vi "sub_scout_cmd-pacekt-conversion.vi"(8 "Frame ID":u8, 10 "Angular Velocity":dbl, 11 "Linear Velocity":dbl) -> (2 "CMD":u8[](array[numeric]))   [LabVIEW 2019]
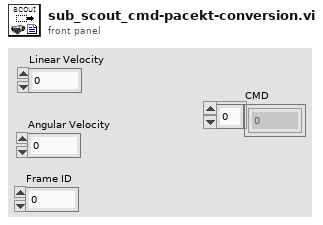
[diagram p1: front panel]
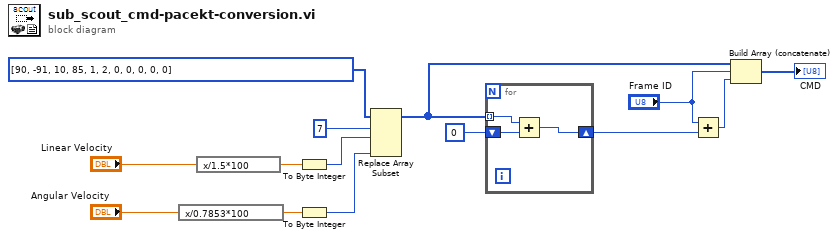
[diagram p0: block diagram]
diagram:
  n1 = expression code="x/0.7853*100"("Angular Velocity") -> (w2:dbl)
  n2 = expression code="x/1.5*100"("Linear Velocity") -> (w5:dbl)
  n3 = To Byte Integer(number=w5) -> (8bit integer=w4:i8)
  n4 = To Byte Integer(number=w2) -> (8bit integer=w1:i8)
  n5 = Replace Array Subset(array=i8[] [90, -91, 10, 85, 1, 2, 0, 0, 0, 0, 0] ("unsigned byte array"), new element #1=w4, index #1=7 ("index"), new element #2=w1) -> (w7:i8[])  [unwired: 1 in]
  n6 = for {
    tunnel: w7 -> [w17] mode=indexing
    shift-right: [w15] -> w13
    shift-left: u8 0 -> [w16]
    n7 = Add(x=w17, y=w16) -> (x+y=w15:u8)
  }
  n8 = Add(x="Frame ID", y=w13) -> (x+y=w11:u8)
  n9 = Build Array (concatenate)(w7, "Frame ID", w11) -> (→"CMD":u8[])
